vi "ROI group-Delete all but first ROI group.vi"(8 "error in (no error)":errorcluster, 9 "Dialogue message type":enum16{"Warning", "Attention"}(ring), 11 "Save? (T)":bool=TRUE) -> (0 "Error out":errorcluster)   [LabVIEW 2013]
uses:
  Typedefs/Group sel cluster.ctl
  Experiment header interface/Typedefs/Save-Load-Save as-Load last enum.ctl
  Global variables/gl_Functional Imaging-Global variables.vi
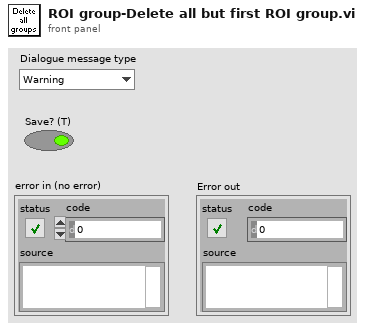
[diagram p1: front panel]
types:
  T1 = typedef "Group sel cluster.ctl" = cluster{"Group number":string, "Group Name":string, "Visibility":bool, "Highlight":bool}
  T2 = typedef "Save-Load-Save as-Load last enum.ctl" = enum16{"Save file", "Save file as", "Load file", "Load last file"}
  T3 = typedef "Functional Imging UI Refs.ctl" = cluster{"Menu ref":refnum<k9>, "Image control":refnum<vi>, "VI ref":refnum<vi>, "XGrapher":refnum<vi>, "Smoothing":refnum<vi>, "POI Averaging":refnum<vi>, "Normalize":refnum<vi>, "POI data points in each trial":refnum<vi>, "Channel":refnum<vi>, "Experiment data folder path":refnum<vi>, "[ROI vis]":refnum<vi>, "[Groups] visbl":T4, "Group Name":refnum<vi>, "POI index":refnum<vi>, "Trial No.":refnum<vi>, "Intensity Zoom":refnum<vi>, "Trial Cursor Enabled":refnum<vi>, "Number of Trials (ind 1)":refnum<vi>, "Number of Trials (ind 2)":refnum<vi>, "MiniScans Available":refnum<vi>, "POI Available":refnum<vi>, "Defer graph updates":refnum<vi>, "Waveform selector":refnum<vi>, "#of selected POI":refnum<vi>, "#of selected MiniScans":refnum<vi>, "#of selected groups":refnum<vi>, "Max Z-Projection":refnum<vi>, "Z-Plane Selector":refnum<vi>, "Index of miniscan point to visualise":refnum<vi>, "ROI vis. mode":refnum<vi>, "Total # of points":refnum<vi>, "Index of group clicked on":refnum<vi>, "Pane 1":refnum<vi>, "Pane 2":refnum<vi>, "Pane 3":refnum<vi>, "Pane 4":refnum<vi>, "Pane 5":refnum<vi>, "Pane 6":refnum<vi>, "Deselect all ROI":refnum<vi>, "Deselect all groups":refnum<vi>}
  T4 = typedef "Groups array referecne.ctl" = refnum<vi>
  T5 = typedef "ROI group info cluster.ctl" = cluster{"Group name":string, "# ROI in group":i32, "ROI numbers in group":i32[], "Group region specifier cluster":T6}
  T6 = typedef "ROI Descriptor" = cluster{"Global Rectangle":i32[], "Contours":cluster{"ID":enum32{"External", "Internal"}, "Type":u32, "Coordinates":i32[]}[]}
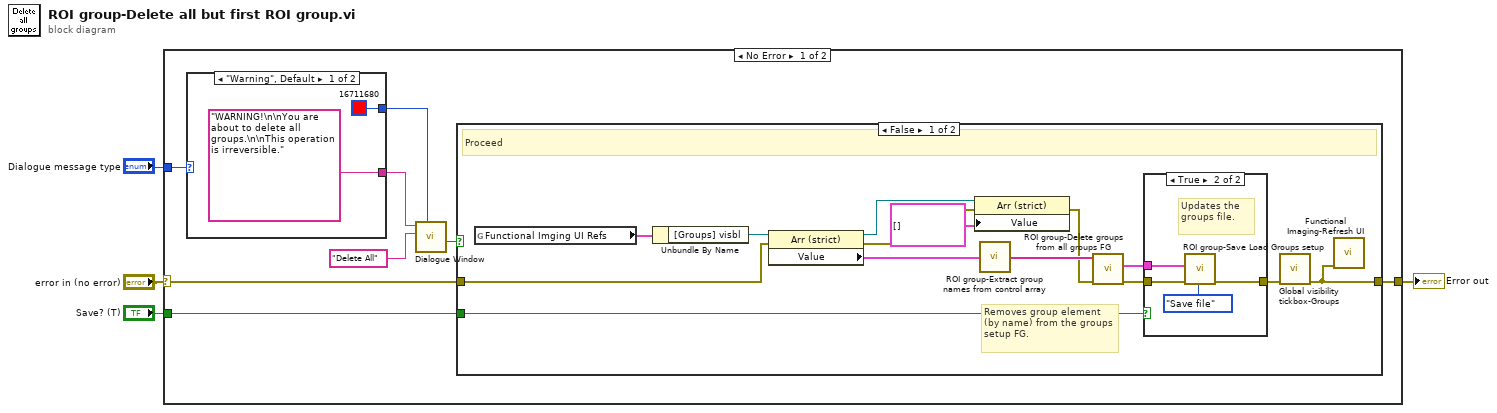
[diagram p0: block diagram]
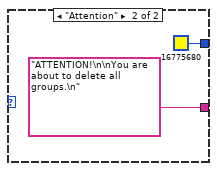
[diagram p2: hidden frame]
diagram:
  n1 = case shown="No Error" "error in (no error)" {
    selector: "error in (no error)" -> [w12 w37]
    tunnel: [w9 w37] -> w3
    tunnel: "Save? (T)" -> [w8 _]
    tunnel: "Dialogue message type" -> [w5 _]
    frame No Error {
      n2 = case shown="\"Warning\", Default" w5 {
        tunnel: ["WARNING!\n\nYou are about to delete all groups.\n\nThis operation is irreversible." ("Message string") "ATTENTION!\n\nYou are about to delete all groups.\n" ("Message string")] -> w7
        tunnel: [u32 16711680 ("Colour") u32 16775680 ("Colour")] -> w6
        frame "Warning", Default {
        }
        frame "Attention" {
        }
      }
      n3 = call "Dialogue Window.vi"("Colour"=w6, "Caption-Right button (OK)"="Delete All", "Message string"=w7) -> ("Cancelled (Left button pressed)"=w11:bool)  [unwired: 6 in, 2 out]
      n4 = case shown="False" w11 {
        tunnel: w12 -> [w21 w36]
        tunnel: [w17 w36] -> w9
        tunnel: w8 -> [w19 _]
        frame False {
          # "Removes group element (by name) from the groups setup FG."
          # "Proceed"
          n5 = global read "gl_Functional Imaging-Global variables.vi" "Functional Imging UI Refs"() -> (w26:T3)
          n6 = Unbundle By Name(w26) -> ("[Groups] visbl"=w27:T4)
          n7 = property on="Property Node" class="Arr (strict)"(reference=w27, error in=w21) -> (reference out=w24:T4, error out=w22:errorcluster, "Value"=w25:T1[])
          n8 = property on="Property Node" class="Arr (strict)"(reference=w24, error in=w22, "Value"=T1[] []) -> (error out=w20:errorcluster)  [unwired: 1 out]
          n9 = call "ROI group-Extract group names from control array.vi"("Groups"=w25) -> ("Group Names Array"=w28:string[])
          n10 = call "ROI group-Delete groups from all groups FG.vi"("error in (no error)"=w20, "Names of groups to delete"=w28) -> ("error out"=w30:errorcluster, "Updated groups setup"=w29:T5[])  [unwired: 8 in]
          n11 = case shown="True" w19 {
            tunnel: w30 -> [w31 w34]
            tunnel: w29 -> [_ w33]
            tunnel: [w31 w32] -> w18
            frame False {
            }
            frame True {
              # "Updates the groups file."
              n12 = call "ROI group-Save Load Groups setup.vi"("error in (no error)"=w34, "Function"=Save-Load-Save_as-Load_last_enum."Save file", "Groups setup to save"=w33) -> ("error out"=w32:errorcluster)  [unwired: 7 in, 1 out]
            }
          }
          n13 = call "Global visibility tickbox-Groups.vi"("error in (no error)"=w18) -> ("error out"=w17:errorcluster)  [unwired: 10 in]
          n14 = call "Functional Imaging-Refresh UI.vi"("error in (no error)"=w17) -> ()  [unwired: 11 in]
        }
        frame True {
          # "Cancelled"
        }
      }
    }
    frame Error {
    }
  }
  "Error out" <- w3
